vi "SystemSNF.vi"() -> ()   [LabVIEW 2017]
uses:
  <vilib>/Analysis/baseanly.llb/Mean (DBL).vi
  <vilib>/Utility/file.llb/Read Delimited Spreadsheet (string).vi
  <vilib>/Utility/file.llb/Write Delimited Spreadsheet (string).vi
  <vilib>/Utility/file.llb/Read Delimited Spreadsheet (DBL).vi
  <vilib>/Utility/file.llb/Write Delimited Spreadsheet (DBL).vi
  <resource>/objmgr/ni.dex.rc
  <vilib>/Analysis/NI_AALBase.lvlib
panel:
  out "System Safe":bool
  in  "Exit Profile":bool
  in  "Select Operation Mode":T1(ring) caption="Select Operation Mode2"
  in  "CTAH Frequency\n[10*Hz]":u16
  in  "CTAH Outlet Set-Point [C]":dbl
  out "System Time [s]":sgl
  out "System Loop Time (ms)":u32
  in  "Pump Mass Flow Set-Point [kg/s]":dbl
  in  "Load Power Profile":bool
  in  "Dyn. Power Profile File":path
  out "CTAH Temperatures":T2(graph)
  out "CTAH Outlet":dbl format="%0.2f"
  out "CTAH Inlet":dbl format="%0.2f"
  out "Core Temperatures":T2(graph)
  out "Heater Outlet":dbl format="%0.2f"
  out "Heater Inlet":dbl format="%0.2f"
  out "Core Power":T2(graph)
  out "FM-60 [kg/s]":sgl
  out "FM-40 [kg/s]":sgl
  out "FM-30 [kg/s]":sgl
  out "FM-20 [kg/s]":sgl
  in  "Tab Control":enum32{"Thermocouple Readings [C]"}(tab)
  out "WT-10":sgl
  out "BT-11":sgl
  out "BT-12":sgl
  out "WT-13":sgl
  out "CX-10":dbl format="%0.2f"
  out "CX-11":dbl format="%0.2f"
  out "WT-20":sgl
  out "BT-21":sgl
  out "WT-22":sgl
  out "BT-23":sgl
  out "WT-24":sgl
  out "BT-25":sgl
  out "WT-26":sgl
  out "BT-27":sgl
  out "WT-28":sgl
  out "BT-29":sgl
  out "BT-30":sgl
  out "WT-31":sgl
  out "BT-32":sgl
  out "WT-33":sgl
  out "BT-34":sgl
  out "WT-35":sgl
  out "WT-40":sgl
  out "BT-41":sgl
  out "WT-42":sgl
  out "BT-43":sgl
  out "BT-60":sgl
  out "WT-61":sgl
  out "WT-62":sgl
  out "BT-63":sgl
  out "WT-64":sgl
  out "BT-65":sgl
  out "BT-66":sgl
  out "WT-67":sgl
  out "ST-10":sgl
  out "ST-11":sgl
  out "ST-12":sgl[](array[numeric])
  out "ST-13":sgl
  out "ST-14":sgl[](array[numeric])
  out "AT-01":sgl
  out "AT-02":sgl
  out "Profile Step":i32
  out "Power Output [W]":dbl
  out "Power Input Signal [W]":dbl
  out "Output Current 2 [A]":dbl
  out "Output Voltage 2 [V]":dbl
  out "Output Current 1 [A]":dbl
  out "Output Voltage 1 [V]":dbl
  out "Loop Period [ms]":i64
  in  "Shutdown":bool
  in  "Desired Power [W]":dbl
  in  "Power Output On":bool
  in  "Pump Frequency\n[10*Hz]":u16
  in  "ACTIVATE - PUMP":bool
  in  "Pump Operation Mode":i32(listbox)
  in  "TCHX Frequency\n[10*Hz]":u16
  in  "ACTIVATE - TCHX":bool
  in  "TCHX Operation Mode":i32(listbox)
  in  "GS1 Stop":bool
  in  "ACTIVATE - CTAH":bool
  in  "CTAH Operation Mode":i32(listbox)
  in  "Error In":errorcluster
  out "Number of Disconnections":u32
  out "Available Elements for Reading":i32
  out "DAQ?":bool
  in  "Stop DAQ":bool
  out "Error Out":errorcluster
  # ".csv file with single column\nAssume constant loop frequency (1 Hz)"
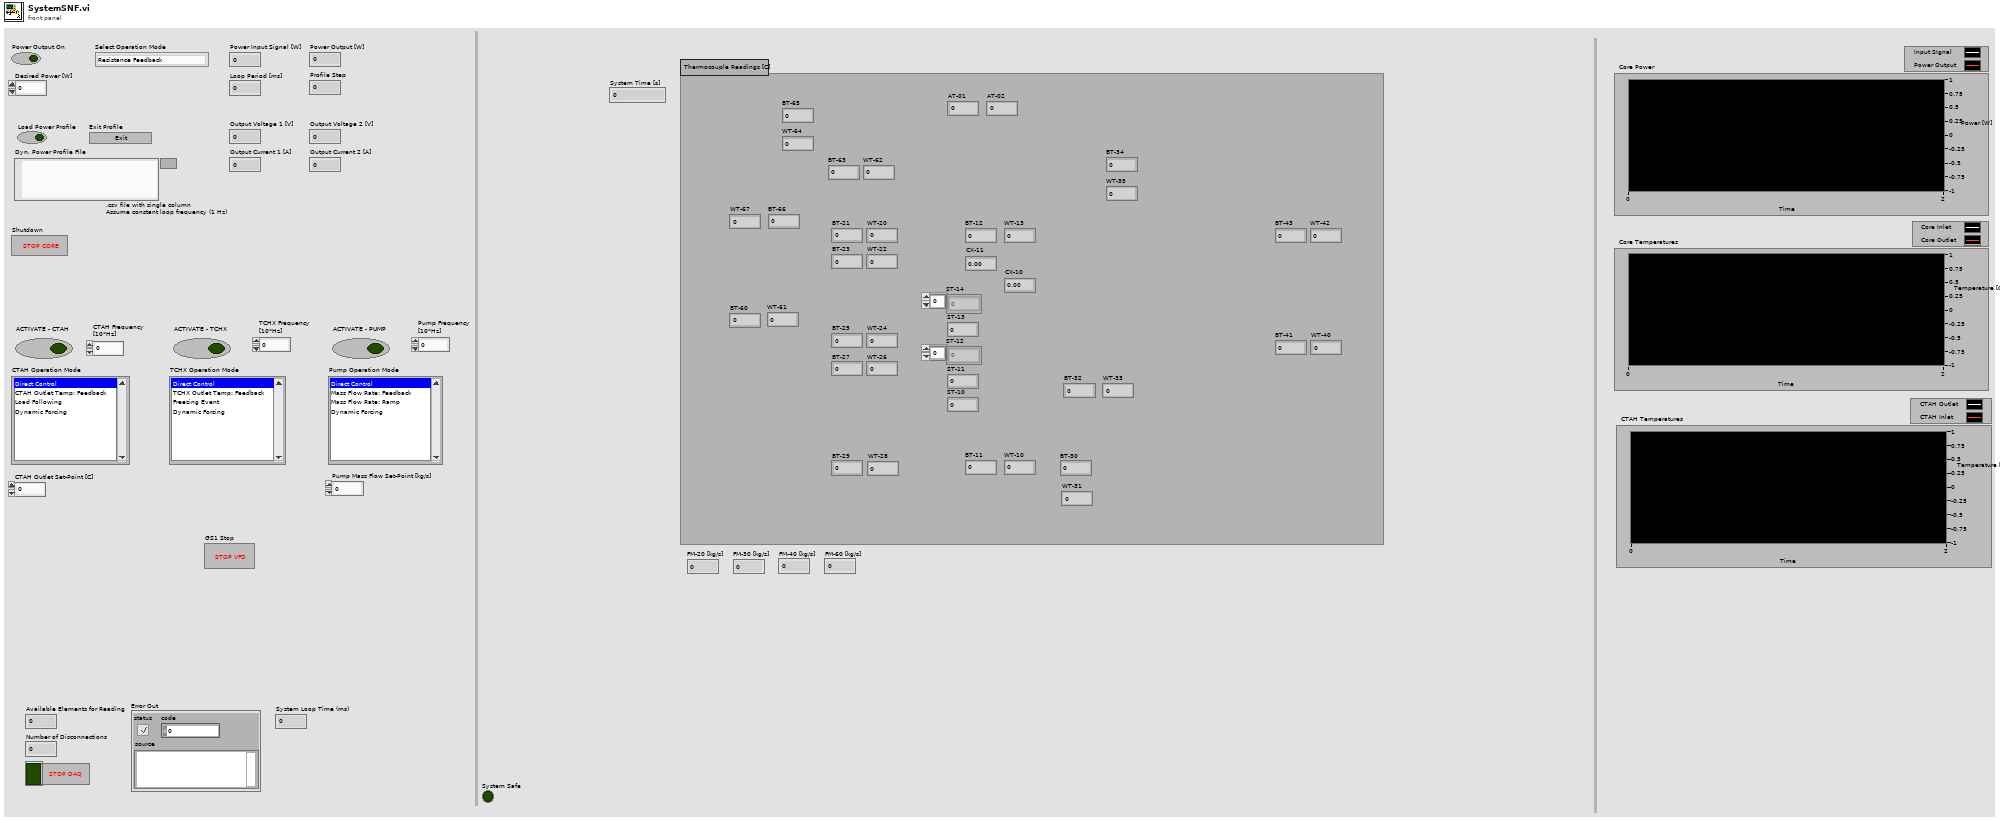
[diagram p1: front panel]
types:
  T1 = enum16{"Resistance Feedback", "Power Profile Input", "Resistance Feedback_Analog", "Power Profile Input_Analog", "Shutdown"}
  T2 = cluster{"Power Input Signal":dbl, "Power Output":dbl}
  T3 = cluster{"Power Input Signal [W]":dbl, "Power Output [W]":dbl}
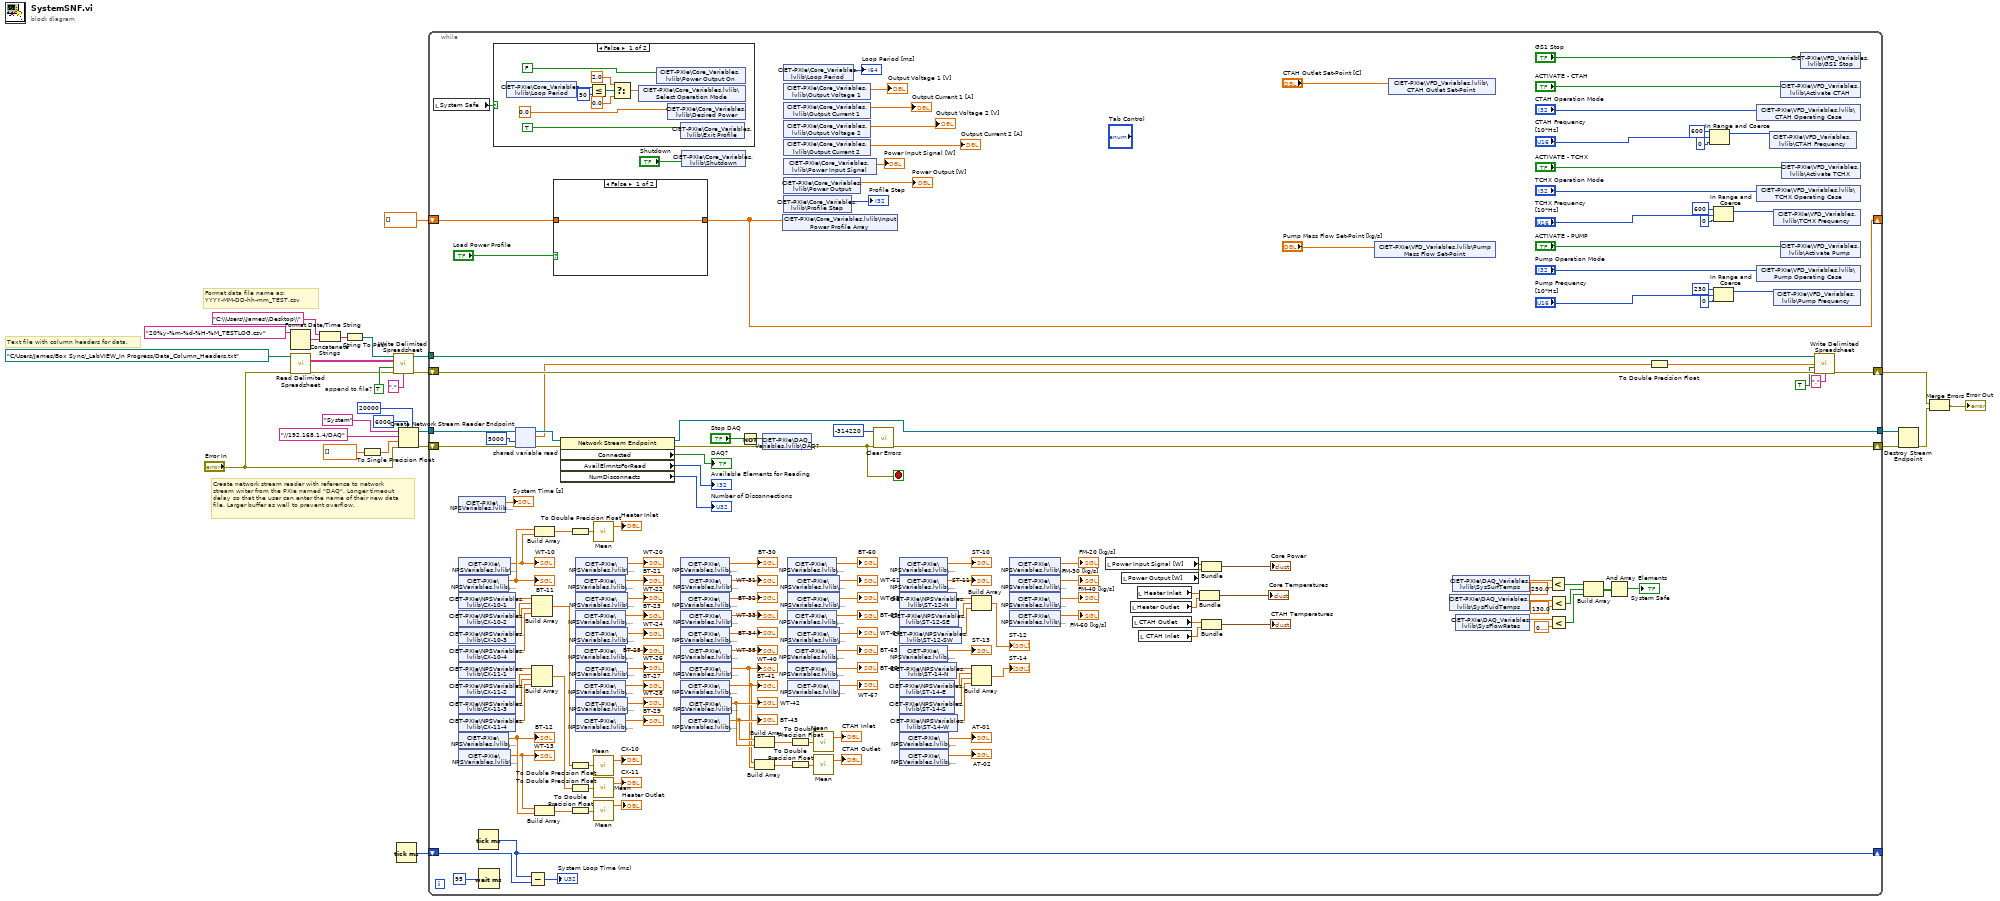
[diagram p0: block diagram]
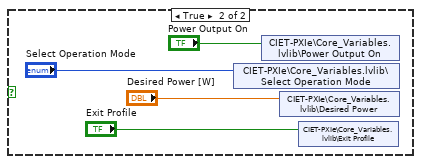
[diagram p2: hidden frame]
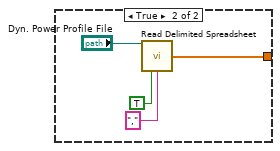
[diagram p3: hidden frame]
diagram:
  w15 = TRUE  # append to file?
  # "Format data file name as:\nYYYY-MM-DD-hh-mm_TEST.csv"
  # "Create network stream reader with reference to network\nstream writer from the PXIe named \"DAQ\". Longer timeout\ndelay so that the user can enter the name of their new data\nfile. Larger buffer as well to prevent overflow."
  # "Text file with column headers for data."
  n1 = Format Date/Time String(time format string (%c)="20%y-%m-%d-%H-%M_TESTLOG.csv") -> (date/time string=w5:string)  [unwired: 2 in]
  n2 = call-poly <vilib>:"Read Delimited Spreadsheet.vi"("file path (dialog if empty)"=path "C:/Users/James/Box Sync/_LabVIEW_In Progress/Data_Column_Headers.txt", "error in (no error)"="Error In") -> ("all rows"=w18:string[][], "error out"=w13:errorcluster)  [unwired: 8 in, 4 out]
  n3 = Concatenate Strings("C:\\Users\\James\\Desktop\\" ("string"), w5) -> (w7:string)
  n4 = String To Path(string=w7) -> (path=w4:path)
  n5 = To Single Precision Float(number=dbl[] []) -> (single precision float=w26:sgl[])
  n6 = call-poly <vilib>:"Write Delimited Spreadsheet.vi"("file path (dialog if empty)"=w4, "2D data"=w18, "append to file? (new file:F)"=w15, "error in (no error)"=w13, "delimiter (\\t)"=",") -> ("new file path (Not A Path if cancelled)"=w14:path, "error out"=w12:errorcluster)  [unwired: 9 in]
  n7 = Tick Count (ms)() -> (millisecond timer value=w1:u32)
  n8 = Create Network Stream Reader Endpoint(5:20000 ("timeout in ms (-1)"), 7:6000 ("reader buffer size"), 8:"Error In", 9:w26, 10:"//192.168.1.4/DAQ" ("writer url"), 11:"System" ("reader name")) -> (0:w23:errorcluster, 3:w22:refnum<k21>)  [unwired: 1 in]
  n9 = while {
    shift-right: [w174] -> w21
    shift-left: w23 -> [w182]
    tunnel: w22 -> [w183]
    tunnel: [w173] -> w20
    tunnel: w14 -> [w169]
    shift-right: [w167] -> w11
    shift-left: w12 -> [w168]
    shift-right: [w53] -> _
    shift-left: dbl[] [] ("Input Power Profile Array") -> [w54]
    shift-right: [w49] -> _
    shift-left: w1 -> [w50]
    stop <- w172 stop-if-true
    n10 = local read "System Safe"() -> (w30:bool)
    n11 = shared-variable "CIET-PXIe\\NPSVariables.lvlib\\Time"() -> (→"System Time [s]":sgl)  [unwired: 1 in, 1 out]
    n12 = shared-variable "CIET-PXIe\\NPSVariables.lvlib\\WT-10"() -> (w74:sgl)  [unwired: 1 in, 1 out]
    "WT-10" <- w74
    n13 = shared-variable "CIET-PXIe\\NPSVariables.lvlib\\BT-11"() -> (w75:sgl)  [unwired: 1 in, 1 out]
    "BT-11" <- w75
    n14 = shared-variable "CIET-PXIe\\NPSVariables.lvlib\\CX-10-1"() -> (w140:sgl)  [unwired: 1 in, 1 out]
    n15 = shared-variable "CIET-PXIe\\NPSVariables.lvlib\\CX-10-2"() -> (w139:sgl)  [unwired: 1 in, 1 out]
    n16 = shared-variable "CIET-PXIe\\NPSVariables.lvlib\\CX-10-3"() -> (w138:sgl)  [unwired: 1 in, 1 out]
    n17 = shared-variable "CIET-PXIe\\NPSVariables.lvlib\\CX-10-4"() -> (w137:sgl)  [unwired: 1 in, 1 out]
    n18 = shared-variable "CIET-PXIe\\NPSVariables.lvlib\\CX-11-1"() -> (w133:sgl)  [unwired: 1 in, 1 out]
    n19 = shared-variable "CIET-PXIe\\NPSVariables.lvlib\\CX-11-2"() -> (w132:sgl)  [unwired: 1 in, 1 out]
    n20 = shared-variable "CIET-PXIe\\NPSVariables.lvlib\\CX-11-3"() -> (w131:sgl)  [unwired: 1 in, 1 out]
    n21 = shared-variable "CIET-PXIe\\NPSVariables.lvlib\\CX-11-4"() -> (w130:sgl)  [unwired: 1 in, 1 out]
    n22 = shared-variable "CIET-PXIe\\NPSVariables.lvlib\\BT-12"() -> (w79:sgl)  [unwired: 1 in, 1 out]
    "BT-12" <- w79
    n23 = shared-variable "CIET-PXIe\\NPSVariables.lvlib\\WT-13"() -> (w78:sgl)  [unwired: 1 in, 1 out]
    "WT-13" <- w78
    n24 = Tick Count (ms)() -> (millisecond timer value=w49:u32)
    n25 = Wait (ms)(milliseconds to wait=u32 95) -> ()  [unwired: 1 out]
    n26 = case shown="False" w30 {
      frame False {
        n27 = shared-variable "CIET-PXIe\\Core_Variables.lvlib\\Loop Period"() -> (w190:i64)  [unwired: 1 in, 1 out]
        n28 = Less Or Equal?(x=w190, y=i64 50) -> (x <= y?=w191:bool)
        n29 = Select(t=2.0, s=w191, f=0.0) -> (s? t:f=w186:dbl)
        n30 = shared-variable "CIET-PXIe\\Core_Variables.lvlib\\Select Operation Mode"(w186) -> ()  [unwired: 1 in, 1 out]
        n31 = shared-variable "CIET-PXIe\\Core_Variables.lvlib\\Power Output On"(FALSE ("Power Output On")) -> ()  [unwired: 1 in, 1 out]
        n32 = shared-variable "CIET-PXIe\\Core_Variables.lvlib\\Desired Power"(0.0 ("Desired Power")) -> ()  [unwired: 1 in, 1 out]
        n33 = shared-variable "CIET-PXIe\\Core_Variables.lvlib\\Exit Profile"(TRUE ("Exit Profile")) -> ()  [unwired: 1 in, 1 out]
      }
      frame True {
        n34 = shared-variable "CIET-PXIe\\Core_Variables.lvlib\\Select Operation Mode"("Select Operation Mode") -> ()  [unwired: 1 in, 1 out]
        n35 = shared-variable "CIET-PXIe\\Core_Variables.lvlib\\Power Output On"("Power Output On") -> ()  [unwired: 1 in, 1 out]
        n36 = shared-variable "CIET-PXIe\\Core_Variables.lvlib\\Desired Power"("Desired Power [W]") -> ()  [unwired: 1 in, 1 out]
        n37 = shared-variable "CIET-PXIe\\Core_Variables.lvlib\\Exit Profile"("Exit Profile") -> ()  [unwired: 1 in, 1 out]
      }
    }
    n38 = shared-variable-read(w183, w182, 5000 ("timeout ms (-1)")) -> (w179:refnum<k21>, w177:errorcluster, w141:sgl[])  [unwired: 1 out]
    n39 = Subtract(x=w49, y=w50) -> (x-y=→"System Loop Time (ms)":u32)
    n40 = Build Array(w140, w139, w138, w137) -> (w136:sgl[])
    n41 = Build Array(w133, w132, w131, w130) -> (w129:sgl[])
    n42 = Build Array(w75, w74) -> (w76:sgl[])
    n43 = Build Array(w78, w79) -> (w80:sgl[])
    n44 = case shown="False" "Load Power Profile" {
      tunnel: [w199 w200] -> w53
      tunnel: w54 -> [w199 _]
      frame False {
      }
      frame True {
        n45 = call-poly <vilib>:"Read Delimited Spreadsheet.vi"("file path (dialog if empty)"="Dyn. Power Profile File", "transpose? (F)"=TRUE, "delimiter (\\t)"="," ("delimiter (\\t)")) -> ("first row"=w200:dbl[])  [unwired: 7 in, 5 out]
      }
    }
    n46 = property class="Network Stream Endpoint"(reference=w179, error in=w177) -> (reference out=w173:refnum<k21>, error out=w178:errorcluster, "Connected"=→"DAQ?":bool, "AvailElmntsForRead"=→"Available Elements for Reading":i32, "NumDisconnects"=→"Number of Disconnections":u32)
    n47 = To Double Precision Float(number=w76) -> (double precision float=w77:dbl[])
    n48 = To Double Precision Float(number=w136) -> (double precision float=w135:dbl[])
    n49 = To Double Precision Float(number=w129) -> (double precision float=w134:dbl[])
    n50 = To Double Precision Float(number=w80) -> (double precision float=w81:dbl[])
    n51 = shared-variable "CIET-PXIe\\NPSVariables.lvlib\\WT-20"() -> (→"WT-20":sgl)  [unwired: 1 in, 1 out]
    n52 = shared-variable "CIET-PXIe\\NPSVariables.lvlib\\BT-21"() -> (→"BT-21":sgl)  [unwired: 1 in, 1 out]
    n53 = shared-variable "CIET-PXIe\\NPSVariables.lvlib\\WT-22"() -> (→"WT-22":sgl)  [unwired: 1 in, 1 out]
    n54 = shared-variable "CIET-PXIe\\NPSVariables.lvlib\\BT-23"() -> (→"BT-23":sgl)  [unwired: 1 in, 1 out]
    n55 = shared-variable "CIET-PXIe\\NPSVariables.lvlib\\WT-24"() -> (→"WT-24":sgl)  [unwired: 1 in, 1 out]
    n56 = shared-variable "CIET-PXIe\\NPSVariables.lvlib\\BT-25"() -> (→"BT-25":sgl)  [unwired: 1 in, 1 out]
    n57 = shared-variable "CIET-PXIe\\NPSVariables.lvlib\\WT-26"() -> (→"WT-26":sgl)  [unwired: 1 in, 1 out]
    n58 = shared-variable "CIET-PXIe\\NPSVariables.lvlib\\BT-27"() -> (→"BT-27":sgl)  [unwired: 1 in, 1 out]
    n59 = shared-variable "CIET-PXIe\\NPSVariables.lvlib\\WT-28"() -> (→"WT-28":sgl)  [unwired: 1 in, 1 out]
    n60 = shared-variable "CIET-PXIe\\NPSVariables.lvlib\\BT-29"() -> (→"BT-29":sgl)  [unwired: 1 in, 1 out]
    n61 = call-poly <vilib>:"Mean.vi"("X"=w77) -> ("mean"=→"Heater Inlet":dbl)  [unwired: 1 out]
    n62 = call-poly <vilib>:"Mean.vi"("X"=w135) -> ("mean"=→"CX-10":dbl)  [unwired: 1 out]
    n63 = call-poly <vilib>:"Mean.vi"("X"=w134) -> ("mean"=→"CX-11":dbl)  [unwired: 1 out]
    n64 = call-poly <vilib>:"Mean.vi"("X"=w81) -> ("mean"=→"Heater Outlet":dbl)  [unwired: 1 out]
    n65 = shared-variable "CIET-PXIe\\NPSVariables.lvlib\\BT-30"() -> (→"BT-30":sgl)  [unwired: 1 in, 1 out]
    n66 = shared-variable "CIET-PXIe\\NPSVariables.lvlib\\WT-31"() -> (→"WT-31":sgl)  [unwired: 1 in, 1 out]
    n67 = shared-variable "CIET-PXIe\\NPSVariables.lvlib\\BT-32"() -> (→"BT-32":sgl)  [unwired: 1 in, 1 out]
    n68 = shared-variable "CIET-PXIe\\NPSVariables.lvlib\\WT-33"() -> (→"WT-33":sgl)  [unwired: 1 in, 1 out]
    n69 = shared-variable "CIET-PXIe\\NPSVariables.lvlib\\BT-34"() -> (→"BT-34":sgl)  [unwired: 1 in, 1 out]
    n70 = shared-variable "CIET-PXIe\\NPSVariables.lvlib\\WT-35"() -> (→"WT-35":sgl)  [unwired: 1 in, 1 out]
    n71 = shared-variable "CIET-PXIe\\NPSVariables.lvlib\\WT-40"() -> (w60:sgl)  [unwired: 1 in, 1 out]
    "WT-40" <- w60
    n72 = shared-variable "CIET-PXIe\\NPSVariables.lvlib\\BT-41"() -> (w59:sgl)  [unwired: 1 in, 1 out]
    "BT-41" <- w59
    n73 = shared-variable "CIET-PXIe\\NPSVariables.lvlib\\WT-42"() -> (w62:sgl)  [unwired: 1 in, 1 out]
    "WT-42" <- w62
    n74 = shared-variable "CIET-PXIe\\NPSVariables.lvlib\\BT-43"() -> (w61:sgl)  [unwired: 1 in, 1 out]
    "BT-43" <- w61
    n75 = shared-variable "CIET-PXIe\\Core_Variables.lvlib\\Shutdown"("Shutdown") -> ()  [unwired: 1 in, 1 out]
    n76 = Not(x="Stop DAQ") -> (.not. x?=w181:bool)
    n77 = Build Array(w61, w62) -> (w67:sgl[])
    n78 = Build Array(w59, w60) -> (w64:sgl[])
    n79 = shared-variable "CIET-PXIe\\DAQ_Variables.lvlib\\DAQ?"(w181, error in=w178) -> (error out=w172:errorcluster)
    n80 = shared-variable "CIET-PXIe\\Core_Variables.lvlib\\Input Power Profile Array"(w53) -> ()  [unwired: 1 in, 1 out]
    n81 = shared-variable "CIET-PXIe\\Core_Variables.lvlib\\Loop Period"() -> (→"Loop Period [ms]":i64)  [unwired: 1 in, 1 out]
    n82 = shared-variable "CIET-PXIe\\Core_Variables.lvlib\\Output Voltage 1"() -> (→"Output Voltage 1 [V]":dbl)  [unwired: 1 in, 1 out]
    n83 = shared-variable "CIET-PXIe\\Core_Variables.lvlib\\Output Current 1"() -> (→"Output Current 1 [A]":dbl)  [unwired: 1 in, 1 out]
    n84 = shared-variable "CIET-PXIe\\Core_Variables.lvlib\\Output Voltage 2"() -> (→"Output Voltage 2 [V]":dbl)  [unwired: 1 in, 1 out]
    n85 = shared-variable "CIET-PXIe\\Core_Variables.lvlib\\Output Current 2"() -> (→"Output Current 2 [A]":dbl)  [unwired: 1 in, 1 out]
    n86 = shared-variable "CIET-PXIe\\Core_Variables.lvlib\\Power Input Signal"() -> (→"Power Input Signal [W]":dbl)  [unwired: 1 in, 1 out]
    n87 = shared-variable "CIET-PXIe\\Core_Variables.lvlib\\Power Output"() -> (→"Power Output [W]":dbl)  [unwired: 1 in, 1 out]
    n88 = shared-variable "CIET-PXIe\\Core_Variables.lvlib\\Profile Step"() -> (→"Profile Step":i32)  [unwired: 1 in, 1 out]
    n89 = shared-variable "CIET-PXIe\\NPSVariables.lvlib\\BT-60"() -> (→"BT-60":sgl)  [unwired: 1 in, 1 out]
    n90 = shared-variable "CIET-PXIe\\NPSVariables.lvlib\\WT-61"() -> (→"WT-61":sgl)  [unwired: 1 in, 1 out]
    n91 = shared-variable "CIET-PXIe\\NPSVariables.lvlib\\WT-62"() -> (→"WT-62":sgl)  [unwired: 1 in, 1 out]
    n92 = shared-variable "CIET-PXIe\\NPSVariables.lvlib\\BT-63"() -> (→"BT-63":sgl)  [unwired: 1 in, 1 out]
    n93 = shared-variable "CIET-PXIe\\NPSVariables.lvlib\\WT-64"() -> (→"WT-64":sgl)  [unwired: 1 in, 1 out]
    n94 = shared-variable "CIET-PXIe\\NPSVariables.lvlib\\BT-65"() -> (→"BT-65":sgl)  [unwired: 1 in, 1 out]
    n95 = shared-variable "CIET-PXIe\\NPSVariables.lvlib\\BT-66"() -> (→"BT-66":sgl)  [unwired: 1 in, 1 out]
    n96 = shared-variable "CIET-PXIe\\NPSVariables.lvlib\\WT-67"() -> (→"WT-67":sgl)  [unwired: 1 in, 1 out]
    n97 = To Double Precision Float(number=w67) -> (double precision float=w68:dbl[])
    n98 = To Double Precision Float(number=w64) -> (double precision float=w65:dbl[])
    n99 = call-poly <vilib>:"Mean.vi"("X"=w68) -> ("mean"=→"CTAH Inlet":dbl)  [unwired: 1 out]
    n100 = call-poly <vilib>:"Mean.vi"("X"=w65) -> ("mean"=→"CTAH Outlet":dbl)  [unwired: 1 out]
    n101 = call <vilib>:"Clear Errors.vi"("error in (no error)"=w172, "specific error code to clear (0: all)"=-314220) -> ("error out"=w174:errorcluster)  [unwired: 4 in, 1 out]
    n102 = shared-variable "CIET-PXIe\\NPSVariables.lvlib\\ST-10"() -> (→"ST-10":sgl)  [unwired: 1 in, 1 out]
    n103 = shared-variable "CIET-PXIe\\NPSVariables.lvlib\\ST-11"() -> (→"ST-11":sgl)  [unwired: 1 in, 1 out]
    n104 = shared-variable "CIET-PXIe\\NPSVariables.lvlib\\ST-12-N"() -> (w100:sgl)  [unwired: 1 in, 1 out]
    n105 = shared-variable "CIET-PXIe\\NPSVariables.lvlib\\ST-12-SE"() -> (w99:sgl)  [unwired: 1 in, 1 out]
    n106 = shared-variable "CIET-PXIe\\NPSVariables.lvlib\\ST-12-SW"() -> (w98:sgl)  [unwired: 1 in, 1 out]
    n107 = shared-variable "CIET-PXIe\\NPSVariables.lvlib\\ST-13"() -> (→"ST-13":sgl)  [unwired: 1 in, 1 out]
    n108 = shared-variable "CIET-PXIe\\NPSVariables.lvlib\\ST-14-N"() -> (w95:sgl)  [unwired: 1 in, 1 out]
    n109 = shared-variable "CIET-PXIe\\NPSVariables.lvlib\\ST-14-E"() -> (w94:sgl)  [unwired: 1 in, 1 out]
    n110 = shared-variable "CIET-PXIe\\NPSVariables.lvlib\\ST-14-S"() -> (w93:sgl)  [unwired: 1 in, 1 out]
    n111 = shared-variable "CIET-PXIe\\NPSVariables.lvlib\\ST-14-W"() -> (w92:sgl)  [unwired: 1 in, 1 out]
    n112 = shared-variable "CIET-PXIe\\NPSVariables.lvlib\\AT-01"() -> (→"AT-01":sgl)  [unwired: 1 in, 1 out]
    n113 = shared-variable "CIET-PXIe\\NPSVariables.lvlib\\AT-02"() -> (→"AT-02":sgl)  [unwired: 1 in, 1 out]
    n114 = Build Array(w100, w99, w98) -> (→"ST-12":sgl[])
    n115 = Build Array(w95, w94, w93, w92) -> (→"ST-14":sgl[])
    n116 = shared-variable "CIET-PXIe\\NPSVariables.lvlib\\FM-20"() -> (→"FM-20 [kg/s]":sgl)  [unwired: 1 in, 1 out]
    n117 = shared-variable "CIET-PXIe\\NPSVariables.lvlib\\FM-30"() -> (→"FM-30 [kg/s]":sgl)  [unwired: 1 in, 1 out]
    n118 = shared-variable "CIET-PXIe\\NPSVariables.lvlib\\FM-40"() -> (→"FM-40 [kg/s]":sgl)  [unwired: 1 in, 1 out]
    n119 = shared-variable "CIET-PXIe\\NPSVariables.lvlib\\FM-60"() -> (→"FM-60 [kg/s]":sgl)  [unwired: 1 in, 1 out]
    n120 = local read "Power Input Signal [W]"() -> (w84:dbl)
    n121 = local read "Power Output [W]"() -> (w83:dbl)
    n122 = local read "Heater Outlet"() -> (w69:dbl)
    n123 = local read "CTAH Outlet"() -> (w57:dbl)
    n124 = local read "Heater Inlet"() -> (w70:dbl)
    n125 = local read "CTAH Inlet"() -> (w56:dbl)
    n126 = Bundle("Heater Inlet"=w70, "Heater Outlet"=w69) -> (→"Core Temperatures":cluster{"Heater Inlet":dbl, "Heater Outlet":dbl})  [unwired: 1 in]
    n127 = Bundle("Power Input Signal [W]"=w84, "Power Output [W]"=w83) -> (→"Core Power":T3)  [unwired: 1 in]
    n128 = Bundle("CTAH Outlet"=w57, "CTAH Inlet"=w56) -> (→"CTAH Temperatures":cluster{"CTAH Outlet":dbl, "CTAH Inlet":dbl})  [unwired: 1 in]
    n129 = shared-variable "CIET-PXIe\\VFD_Variables.lvlib\\Pump Mass Flow Set-Point"("Pump Mass Flow Set-Point [kg/s]") -> ()  [unwired: 1 in, 1 out]
    n130 = shared-variable "CIET-PXIe\\VFD_Variables.lvlib\\CTAH Outlet Set-Point"("CTAH Outlet Set-Point [C]") -> ()  [unwired: 1 in, 1 out]
    n131 = shared-variable "CIET-PXIe\\DAQ_Variables.lvlib\\SysFluidTemps"() -> (w36:sgl[])  [unwired: 1 in, 1 out]
    n132 = shared-variable "CIET-PXIe\\DAQ_Variables.lvlib\\SysSurfTemps"() -> (w38:sgl[])  [unwired: 1 in, 1 out]
    n133 = shared-variable "CIET-PXIe\\DAQ_Variables.lvlib\\SysFlowRates"() -> (w34:sgl[])  [unwired: 1 in, 1 out]
    n134 = Less?(x=w38, y=sgl 250.0) -> (x < y?=w40:bool[])
    n135 = Less?(x=w36, y=sgl 130.0) -> (x < y?=w33:bool[])
    n136 = Less?(x=w34, y=sgl 0.2) -> (x < y?=w32:bool[])
    n137 = Build Array(w40, w33, w32) -> (w41:bool[][])
    n138 = And Array Elements(Boolean array=w41) -> (logical AND=→"System Safe":bool)
    n139 = To Double Precision Float(number=w141) -> (double precision float=w51:dbl[])
    n140 = In Range and Coerce(upper limit=u16 600, x="CTAH Frequency\n[10*Hz]", lower limit=u16 0) -> (coerced(x)=w45:u16)  [unwired: 1 out]
    n141 = In Range and Coerce(upper limit=u16 600, x="TCHX Frequency\n[10*Hz]", lower limit=u16 0) -> (coerced(x)=w159:u16)  [unwired: 1 out]
    n142 = In Range and Coerce(upper limit=u16 230, x="Pump Frequency\n[10*Hz]", lower limit=u16 0) -> (coerced(x)=w153:u16)  [unwired: 1 out]
    n143 = shared-variable "CIET-PXIe\\VFD_Variables.lvlib\\CTAH Operating Case"("CTAH Operation Mode") -> ()  [unwired: 1 in, 1 out]
    n144 = shared-variable "CIET-PXIe\\VFD_Variables.lvlib\\Pump Operating Case"("Pump Operation Mode") -> ()  [unwired: 1 in, 1 out]
    n145 = shared-variable "CIET-PXIe\\VFD_Variables.lvlib\\TCHX Operating Case"("TCHX Operation Mode") -> ()  [unwired: 1 in, 1 out]
    n146 = shared-variable "CIET-PXIe\\VFD_Variables.lvlib\\CTAH Frequency"(w45) -> ()  [unwired: 1 in, 1 out]
    n147 = shared-variable "CIET-PXIe\\VFD_Variables.lvlib\\Pump Frequency"(w153) -> ()  [unwired: 1 in, 1 out]
    n148 = shared-variable "CIET-PXIe\\VFD_Variables.lvlib\\TCHX Frequency"(w159) -> ()  [unwired: 1 in, 1 out]
    n149 = shared-variable "CIET-PXIe\\VFD_Variables.lvlib\\Activate CTAH"("ACTIVATE - CTAH") -> ()  [unwired: 1 in, 1 out]
    n150 = shared-variable "CIET-PXIe\\VFD_Variables.lvlib\\Activate Pump"("ACTIVATE - PUMP") -> ()  [unwired: 1 in, 1 out]
    n151 = shared-variable "CIET-PXIe\\VFD_Variables.lvlib\\Activate TCHX"("ACTIVATE - TCHX") -> ()  [unwired: 1 in, 1 out]
    n152 = shared-variable "CIET-PXIe\\VFD_Variables.lvlib\\GS1 Stop"("GS1 Stop") -> ()  [unwired: 1 in, 1 out]
    n153 = call-poly <vilib>:"Write Delimited Spreadsheet.vi"("file path (dialog if empty)"=w169, "1D data"=w51, "append to file? (new file:F)"=TRUE, "error in (no error)"=w168, "delimiter (\\t)"="," ("delimiter (\\t)")) -> ("error out"=w167:errorcluster)  [unwired: 9 in, 1 out]
  }
  n154 = Destroy Stream Endpoint(8:w21, 11:w20) -> (0:w10:errorcluster)
  n155 = Merge Errors(w11, w10) -> (→"Error Out":errorcluster)
